vi "sc5511a_open_device.vi"(0 "COM (String) eg COM1":string, 5 "error in (no error)":errorcluster) -> (14 "deviceHandle":u32 format="%.0x", 19 "error out":errorcluster)   [LabVIEW 2010]
uses:
  sc5511a_rs232.dll
panel:
  in  "Baud_rate":enum16{"57600", "115200"}(ring)
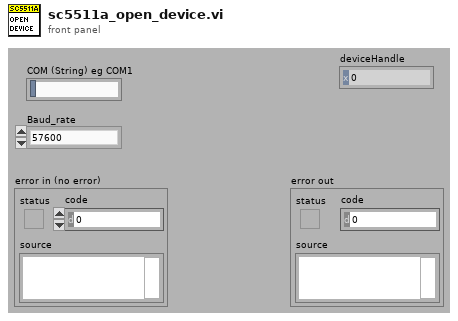
[diagram p1: front panel]
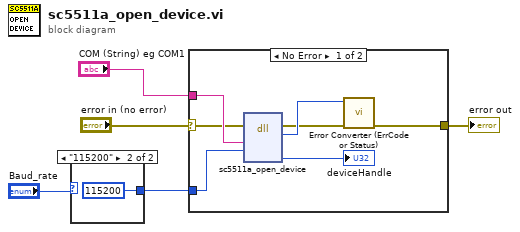
[diagram p0: block diagram]
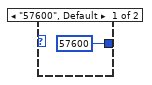
[diagram p2: hidden frame]
diagram:
  n1 = case shown="\"115200\"" "Baud_rate" {
    tunnel: [u32 57600 ("dev_handle") u32 115200 ("dev_handle")] -> w1
    frame "57600", Default {
    }
    frame "115200" {
    }
  }
  n2 = case shown="No Error" "error in (no error)" {
    selector: "error in (no error)" -> [w13 w15]
    tunnel: [w8 w15] -> w4
    tunnel: "COM (String) eg COM1" -> [w14 _]
    tunnel: w1 -> [w10 _]
    frame No Error {
      n3 = dll-call lib="sc5511a_rs232.dll" fn="sc5511a_open_device"(error in=w13, "comm_name"=w14, "baud_rate"=w10) -> (error out=w9:errorcluster, "status"=w12:u32, "dev_handle"=→"deviceHandle":u32)  [unwired: 5 in, 1 out]
      n4 = call "Error Converter (ErrCode or Status).vi"("error in (no error)"=w9, "error code"=w12) -> ("error out"=w8:errorcluster)  [unwired: 9 in]
    }
    frame Error {
    }
  }
  "error out" <- w4
